vi "AddOption_PieTooltips.vi"(0 "reference in":refnum<class "HTMLPlot.lvclass">, 2 "OptionsIn":string[](array[string]), 5 "error in (no error)":errorcluster) -> (14 "reference out":refnum<class "HTMLPlot.lvclass">, 16 "OptionsOut":string[](array[string]), 19 "error out":errorcluster)   [LabVIEW 2019, in "HTMLPlot.lvclass"]
uses:
  HTMLPlot.lvclass
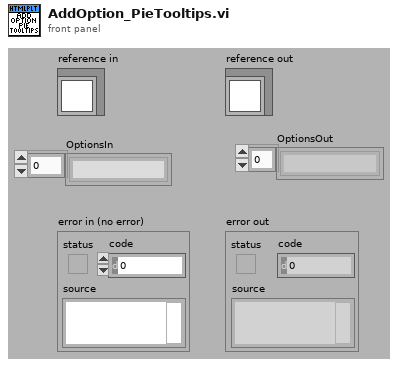
[diagram p1: front panel]
types:
  T1 = typedef "HTMLPlot.lvclass/ObjectAttributes.ctl" = cluster{"Attribute1":dbl, "GraphContainer":refnum<k7>, "ChartScriptFile":string, "UtilScriptFile(demoData)":string, "BaseHTML":string, "GenericProperties":cluster{"PlotType":T2, "PlotTitle":string, "XLabel":string, "YLabel":string, "ShowToolTip":bool}, "LegendProperties":cluster{"Show":bool, "Position":T3}, "BarPlot":cluster{"Dataset":dbl[][], "DatasetLabels":string[], "XLabels":string[], "PlotColours":u32[], "Stacked":bool}, "PiePlot":cluster{"Dataset":dbl[][], "DatasetLabels":string[], "PlotColours":u32[], "DoughnutStyle":bool, "PlotLabels":string[]}, "connection ID":refnum<k5>, "PortID":u64}
  T2 = typedef "HTMLPlot.lvclass/PlotType.ctl" = enum16{"bar", "line", "pie"}
  T3 = typedef "HTMLPlot.lvclass/LegendPosition.ctl" = enum16{"top", "right", "left", "bottom"}
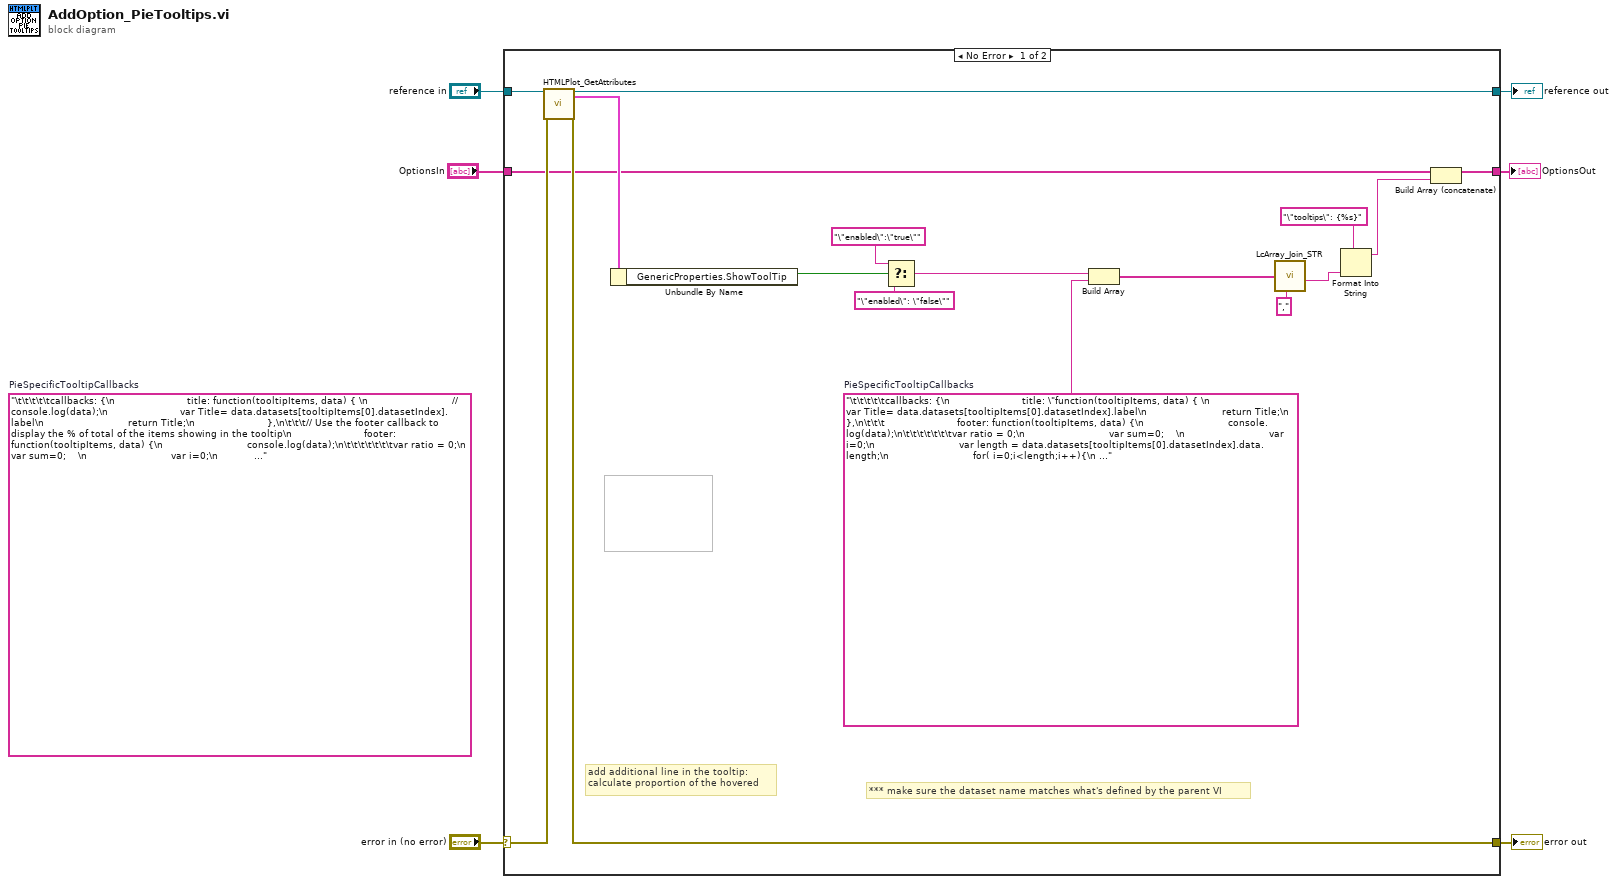
[diagram p0: block diagram]
diagram:
  (unwired) "\t\t\t\t\tcallbacks: {\n                        title: function(tooltipItems, data) { \n                            //console.log(data);\n                        var Title= data.datasets[tooltipItems[0].datasetIndex].label\n                            return Title;\n                        },\n\t\t\t// Use the footer callback to display the % of total of the items showing in the tooltip\n                        footer: function(tooltipItems, data) {\n                            console.log(data);\n\t\t\t\t\t\t\tvar ratio = 0;\n                            var sum=0;    \n                            var i=0;\n                            var length = data.datasets[tooltipItems[0].datasetIndex].data.length;\n                            for( i=0;i<length;i++){\n                                sum+= data.datasets[tooltipItems[0].datasetIndex].data[i];\n                            }\n\t\t\t\t\t\t\ttooltipItems.forEach(function(tooltipItem) {\n\t\t\t\t\t\t\t\tratio = 100*data.datasets[tooltipItem.datasetIndex].data[tooltipItem.index]/sum;\n                                ratio=ratio.toFixed(1)\n\t\t\t\t\t\t\t});\n\t\t\t\t\t\t\treturn 'ratio: ' + ratio + '%' ;\n\t\t\t\t\t\t},\n\t\t\t\t\t},\n\t\t\t\t\tfooterFontStyle: 'normal'"  # PieSpecificTooltipCallbacks
  n1 = case shown="No Error" "error in (no error)" {
    selector: "error in (no error)" -> [w23 w26]
    tunnel: [w21 w26] -> w5
    tunnel: [w19 w25] -> w3
    tunnel: "reference in" -> [w20 w25]
    tunnel: "OptionsIn" -> [w18 w24]
    tunnel: [w17 w24] -> w1
    frame No Error {
      w9 = "\t\t\t\t\tcallbacks: {\n                        title: \"function(tooltipItems, data) { \n                         var Title= data.datasets[tooltipItems[0].datasetIndex].label\n                         return Title;\n                        },\n\t\t\t                        footer: function(tooltipItems, data) {\n                            console.log(data);\n\t\t\t\t\t\t\tvar ratio = 0;\n                            var sum=0;    \n                            var i=0;\n                            var length = data.datasets[tooltipItems[0].datasetIndex].data.length;\n                            for( i=0;i<length;i++){\n                                sum+= data.datasets[tooltipItems[0].datasetIndex].data[i];\n                            }\n\t\t\t\t\t\t\ttooltipItems.forEach(function(tooltipItem) {\n\t\t\t\t\t\t\t\tratio = 100*data.datasets[tooltipItem.datasetIndex].data[tooltipItem.index]/sum;\n                                ratio=ratio.toFixed(1)\n\t\t\t\t\t\t\t});\n\t\t\t\t\t\t\treturn 'ratio: ' + ratio + '%' ;\n\t\t\t\t\t\t},\n\t\t\t\t\t},\n\t\t\t\t\tfooterFontStyle: 'normal'"  # PieSpecificTooltipCallbacks
      # "add additional line in the tooltip:\ncalculate proportion of the hovered"
      # "*** make sure the dataset name matches what's defined by the parent VI"
      n2 = call "HTMLPlot_GetAttributes.vi"("reference in"=w20, "error in (no error)"=w23) -> ("reference out"=w19:refnum<class "HTMLPlot.lvclass">, "Data"=w22:T1, "error out"=w21:errorcluster)  [unwired: 14 in, 1 out]
      n3 = Unbundle By Name(w22) -> ("GenericProperties.ShowToolTip"=w13:bool)
      n4 = Select(t="\"enabled\":\"true\"", s=w13, f="\"enabled\": \"false\"") -> (s? t:f=w10:string)
      n5 = Build Array(w10, w9) -> (w8:string[])
      n6 = call "LcArray_Join_STR.vi"("separator"=",", "Array"=w8) -> ("joined string"=w7:string)  [unwired: 8 in, 1 out]
      n7 = Format Into String(format string="\"tooltips\": {%s}", w7) -> (resulting string=w16:string)  [unwired: 2 in, 1 out]
      n8 = Build Array (concatenate)(w18, w16) -> (w17:string[])
    }
    frame Error {
    }
  }
  "error out" <- w5
  "reference out" <- w3
  "OptionsOut" <- w1
